vi "Actor Core.vi"(8 "error in":errorcluster, 11 "PVClient-Example in":refnum<class "PVClient-Example.lvclass">) -> (0 "error out":errorcluster, 3 "Actor out":refnum<class "Actor.lvclass">)   [LabVIEW 2013, in "PVClient-Example.lvlib" / "PVClient-Example.lvclass"]
doc: "(<B>Filename</B>: Actor Framework.lvlib:Actor.lvclass:Actor Core.vi)\n\nReceives messages to the actor, reacts to them, and initiates any error handling that may shut the actor down.\n\nDescendant classes may override this VI to append parallel tasks for the actor to complete while it handles messages. Overrides use the Call Parent Method node."
uses:
  PVClient-Example.lvclass
  <vilib>/ActorFramework/Actor/Actor.lvclass
  CSPP_Core/Actors/CS++SVMonitor/CS++SVMonitor.lvclass
  PVClient-Example Messages/PVUpdate-myDouble Msg.lvclass
  CSPP_Core/Actors/CS++BaseActor/CS++BaseActor.lvclass/CS++BaseActor.ctl
  <vilib>/ActorFramework/Actor/Actor.lvclass/Actor.ctl
  <vilib>/ActorFramework/Message Enqueuer/Message Enqueuer.lvclass/Message Enqueuer.ctl
  PVClient-Example.lvclass/PVClient-Example.ctl
  CSPP_Core/Actors/CS++PVMonitor/CS++PVMonitor.lvclass/CS++PVMonitor.ctl
  CSPP_Core/Actors/CS++PVMonitor Messages/Register PVs Msg/Register PVs Msg.lvclass/Register PVs Msg.ctl
  CSPP_Core/Actors/CS++BaseActor/CS++BaseActor.lvclass
  <vilib>/ActorFramework/Message Enqueuer/Init from Existing Queue.vi
  <vilib>/ActorFramework/Message Enqueuer/Enqueue.vi
  <vilib>/ActorFramework/Message Priority Queue/Priority Enqueue.vi
  <vilib>/ActorFramework/Message Enqueuer/Message Enqueuer.lvclass
  CSPP_Core/Actors/CS++PVMonitor Messages/Register PVs Msg/Register PVs Msg.lvclass
  <vilib>/ActorFramework/Stop Msg/Stop Msg.lvclass
  CSPP_Core/Actors/CS++PVMonitor/CS++PVMonitor.lvclass
panel:
  out "myDouble":dbl
  in  "Stop Button":bool
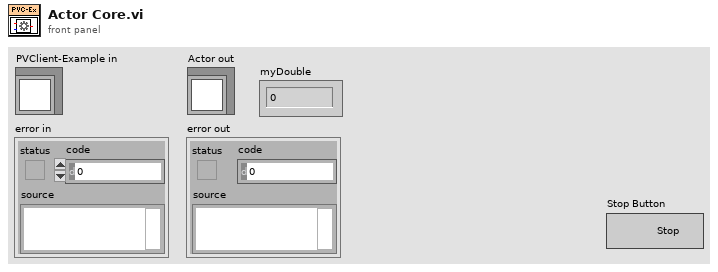
[diagram p1: front panel]
types:
  T1 = enum32{"Invalid", "Standard", "Closed", "Hidden", "Minimized", "Maximized"}
  T2 = cluster{"PV URL":string, "PVClient-Example.lvlib:PVUpdate-myDouble Msg.lvclass":refnum<class "PVUpdate-myDouble Msg.lvclass">}
  T3 = cluster{"PV URL":string, "PVClient-Example.lvlib:PVUpdate-myDouble Msg.lvclass":refnum<class "PVUpdate-myDouble Msg.lvclass">}[]
  T4 = cluster{"Self Enqueuer":refnum<class "Message Enqueuer.lvclass">, cluster{"PV URL":string, "PVClient-Example.lvlib:PVUpdate-myDouble Msg.lvclass":refnum<class "PVUpdate-myDouble Msg.lvclass">}[]}
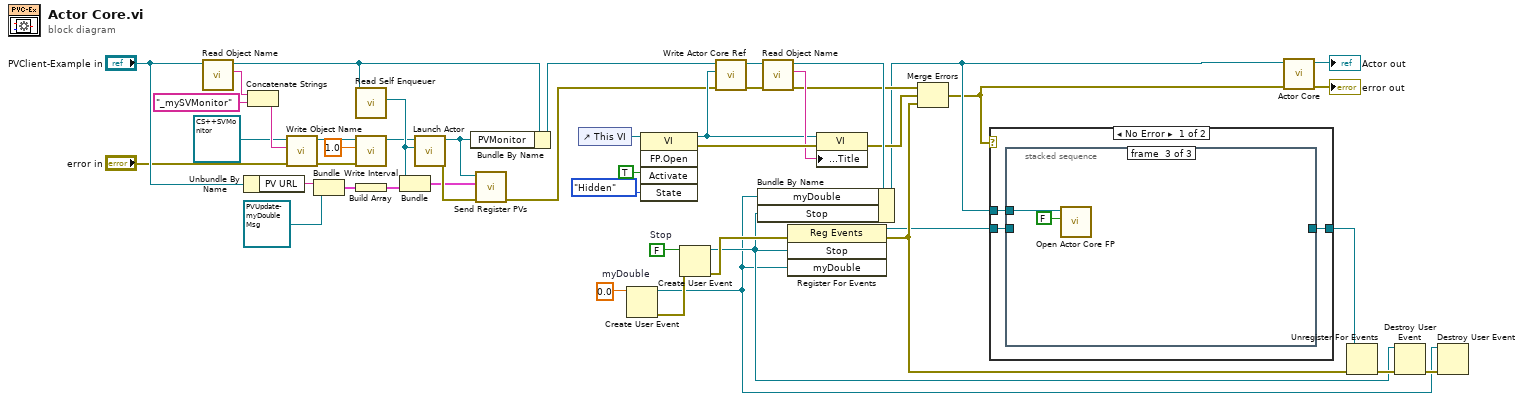
[diagram p0: block diagram]
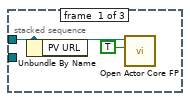
[diagram p2: hidden frame]
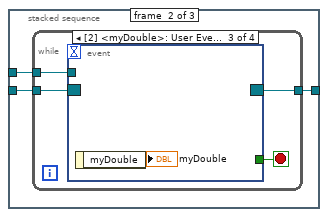
[diagram p3: hidden frame]
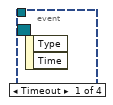
[diagram p4: hidden frame]
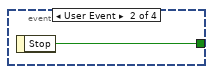
[diagram p5: hidden frame]
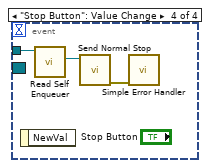
[diagram p6: hidden frame]
diagram:
  w4 = 0.0  # myDouble
  w33 = FALSE  # Stop
  n1 = call "Read Object Name.vi"("CS++BaseActor in"="PVClient-Example in") -> ("Object Name"=w16:string, "CS++BaseActor out"=w17:refnum<class "PVClient-Example.lvclass">)  [unwired: 8 in, 1 out]
  n2 = Unbundle By Name("PVClient-Example in") -> ("PV URL"=w45:string)
  n3 = Concatenate Strings(w16, "_mySVMonitor" ("Object Name")) -> (w12:string)
  n4 = call "Write Object Name.vi"("error in (no error)"="error in", "Object Name"=w12, "CS++BaseActor in"=refnum<class "CS++SVMonitor.lvclass"> refnum ("CS++SVMonitor.lvlib:CS++SVMonitor.lvclass")) -> ("error out"=w8:errorcluster, "CS++BaseActor out"=w11:refnum<class "CS++SVMonitor.lvclass">)  [unwired: 7 in]
  n5 = Bundle("PV URL"=w45, "PVClient-Example.lvlib:PVUpdate-myDouble Msg.lvclass"=refnum<class "PVUpdate-myDouble Msg.lvclass"> refnum) -> (w44:T2)  [unwired: 1 in]
  n6 = call <vilib>:"Read Self Enqueuer.vi"("Actor"=w17) -> ("Self Enqueuer"=w41:refnum<class "Message Enqueuer.lvclass">)  [unwired: 10 in]
  n7 = call "Write Interval.vi"("error in (no error)"=w8, "Interval"=dbl[unit] 1.0, "CS++PVMonitor in"=w11) -> ("CS++PVMonitor out"=w13:refnum<class "CS++SVMonitor.lvclass">)  [unwired: 7 in, 1 out]
  n8 = Build Array(w44) -> (w43:T3)
  n9 = Bundle("Self Enqueuer"=w41, w43) -> (w42:T4)  [unwired: 1 in]
  n10 = call <vilib>:"Launch Actor.vi"("Actor-to-Caller Enqueuer"=w41, "Actor"=w13) -> ("error out"=w47:errorcluster, "Caller-To-Actor Enqueuer"=w46:refnum<class "Message Enqueuer.lvclass">)  [unwired: 8 in]
  n11 = Bundle By Name(cluster=w17, "PVMonitor"=w46) -> (w19:refnum<class "PVClient-Example.lvclass">)
  n12 = call "Send Register PVs.vi"("error in (no error)"=w47, "Register Info"=w42, "Message Enqueuer"=w46) -> ("error out"=w18:errorcluster)  [unwired: 7 in, 1 out]
  n13 = control-ref of="This VI"() -> (w40:refnum<vi>)
  n14 = Create User Event(user event datatype=w4) -> (user event=w1:refnum<user-event>, error out=w5:errorcluster)  [unwired: 1 in]
  n15 = invoke class="VI" method="FP.Open"(reference=w40, "Activate"=TRUE ("Activate?"), "State"=T1."Hidden") -> (reference out=w22:refnum<vi>, error out=w35:errorcluster)  [unwired: 2 in, 3 out]
  n16 = Create User Event(user event datatype=w33, error in=w5) -> (user event=w23:refnum<user-event>, error out=w27:errorcluster)
  n17 = call "Write Actor Core Ref.vi"("error in (no error)"=w18, "Actor Core Ref"=w22, "CS++BaseActor in"=w19) -> ("error out"=w37:errorcluster, "CS++BaseActor out"=w36:refnum<class "PVClient-Example.lvclass">)  [unwired: 7 in]
  n18 = call "Read Object Name.vi"("error in (no error)"=w37, "CS++BaseActor in"=w36) -> ("error out"=w30:errorcluster, "Object Name"=w34:string, "CS++BaseActor out"=w32:refnum<class "PVClient-Example.lvclass">)  [unwired: 7 in]
  n19 = Bundle By Name(cluster=w32, "myDouble"=w1, "Stop"=w23) -> (w29:refnum<class "PVClient-Example.lvclass">)
  n20 = register-events(error in=w27, w23, w1) -> (reference out=w25:refnum<event-registration>, error out=w26:errorcluster)  [unwired: 1 in]
  n21 = property class="VI"(reference=w22, error in=w35, "Front Panel.Title"=w34) -> (error out=w31:errorcluster)  [unwired: 1 out]
  n22 = Merge Errors(w30, w31, w26) -> (w6:errorcluster)
  n23 = case shown="No Error" w6 {
    tunnel: w29 -> [w50 _]
    tunnel: w25 -> [w49 w67]
    tunnel: [w48 w67] -> w24
    frame No Error {
      n24 = stacked-sequence {
        tunnel: w50 -> [w52 w54 w66]
        tunnel: w49 -> [_ w55 _]
        tunnel: [_ w53 _] -> w48
        frame #0 {
          n25 = Unbundle By Name(w52) -> ()  [unwired: 1 out]
          n26 = call "Open Actor Core FP.vi"("Open FP (F)"=TRUE, "CS++BaseActor in"=w52) -> ()  [unwired: 8 in, 2 out]
        }
        frame #1 {
          n27 = while {
            tunnel: w55 -> [w59]
            tunnel: w54 -> [w58]
            tunnel: [w56] -> w53
            stop <- w57 stop-if-true
            n28 = event shown="[2] <myDouble>: User Event" {
              selector: w59 -> [_ _ _ _]
              dyn-events: [_ _ _ _] -> w56
              timeout: _ -> [_ _ _ _]
              tunnel: w58 -> [_ _ _ w64]
              tunnel: [_ w60 _ _] -> w57
              event Timeout {
                n29 = event-data() -> ()  [unwired: 1 in, 2 out]
              }
              event User Event {
                n30 = event-data() -> ("Stop"=w60:bool)  [unwired: 1 in]
              }
              event User Event {
                n31 = event-data() -> ("myDouble"=→"myDouble":dbl)  [unwired: 1 in]
              }
              event "Stop Button": Value Change {
                n32 = event-data() -> ()  [unwired: 1 in, 1 out]
                n33 = call <vilib>:"Read Self Enqueuer.vi"("Actor"=w64) -> ("Self Enqueuer"=w63:refnum<class "Message Enqueuer.lvclass">)  [unwired: 10 in]
                n34 = call <vilib>:"Send Normal Stop.vi"("Message Enqueuer"=w63) -> ("error out"=w62:errorcluster)  [unwired: 10 in]
                n35 = call <vilib>:"Simple Error Handler.vi"("error in (no error)"=w62) -> ()  [unwired: 4 in, 5 out]
              }
            }
          }
        }
        frame #2 {
          n36 = call "Open Actor Core FP.vi"("Open FP (F)"=FALSE, "CS++BaseActor in"=w66) -> ()  [unwired: 8 in, 2 out]
        }
      }
    }
    frame Error {
    }
  }
  n37 = call-parent "Actor Core.vi"("error in"=w6, "CS++BaseActor in"=w29) -> ("error out"=→"error out":errorcluster, "Actor out"=→"Actor out":refnum<class "Actor.lvclass">)  [unwired: 8 in]
  n38 = Unregister For Events(event registration refnum=w24, error in=w26) -> (error out=w28:errorcluster)
  n39 = Destroy User Event(user event=w23, error in=w28) -> (error out=w3:errorcluster)
  n40 = Destroy User Event(user event=w1, error in=w3) -> ()  [unwired: 1 out]
